vi "merge-array-teste.vi"() -> ()   [LabVIEW 2014]
panel:
  out "output array":dbl[][](array[numeric])=[[49229.86363636363, 160793.81818181818, 459.7801430124, 626.2382997563999, 1419.6569638843712, 2545.9781193333406, 0.005163496779999999], [49166.0, 160790.5, 459.7801430124, 626.2382997563999, 1416.8691367377512, 2555.19013913818, 0.005163496779999999], [48661.068181818184, 159414.9659090909, 459.7801430124, 626.2382997563999, 1394.3056048740445, 2530.385783266425, 0.005163496779999999], [48702.0, 159927.9, 459.7801430124, 626.9865226475, 1405.3506776205356, 2522.9374551760125, 0.005163496779999999], [49455.07575757576, 161404.96212121213, 459.7801430124, 626.2382997563999, 1427.5985476418132, 2551.9671860210565, 0.005163496779999999]]
  in  "Power Meter":dbl[](array[numeric])=[0.005163496779999999, 0.005163496779999999, 0.005163496779999999, 0.005163496779999999, 0.005163496779999999]
  in  "Amplitudes":dbl[][](array[numeric])=[[1419.6569638843712, 2545.9781193333406], [1416.8691367377512, 2555.19013913818], [1394.3056048740445, 2530.385783266425], [1405.3506776205356, 2522.9374551760125], [1427.5985476418132, 2551.9671860210565]]
  in  "Locations Peaks":dbl[][](array[numeric])=[[459.7801430124, 626.2382997563999], [459.7801430124, 626.2382997563999], [459.7801430124, 626.2382997563999], [459.7801430124, 626.9865226475], [459.7801430124, 626.2382997563999]]
  in  "Integration":dbl[][](array[numeric])=[[49229.86363636363, 160793.81818181818], [49166.0, 160790.5], [48661.068181818184, 159414.9659090909], [48702.0, 159927.9], [49455.07575757576, 161404.96212121213]]
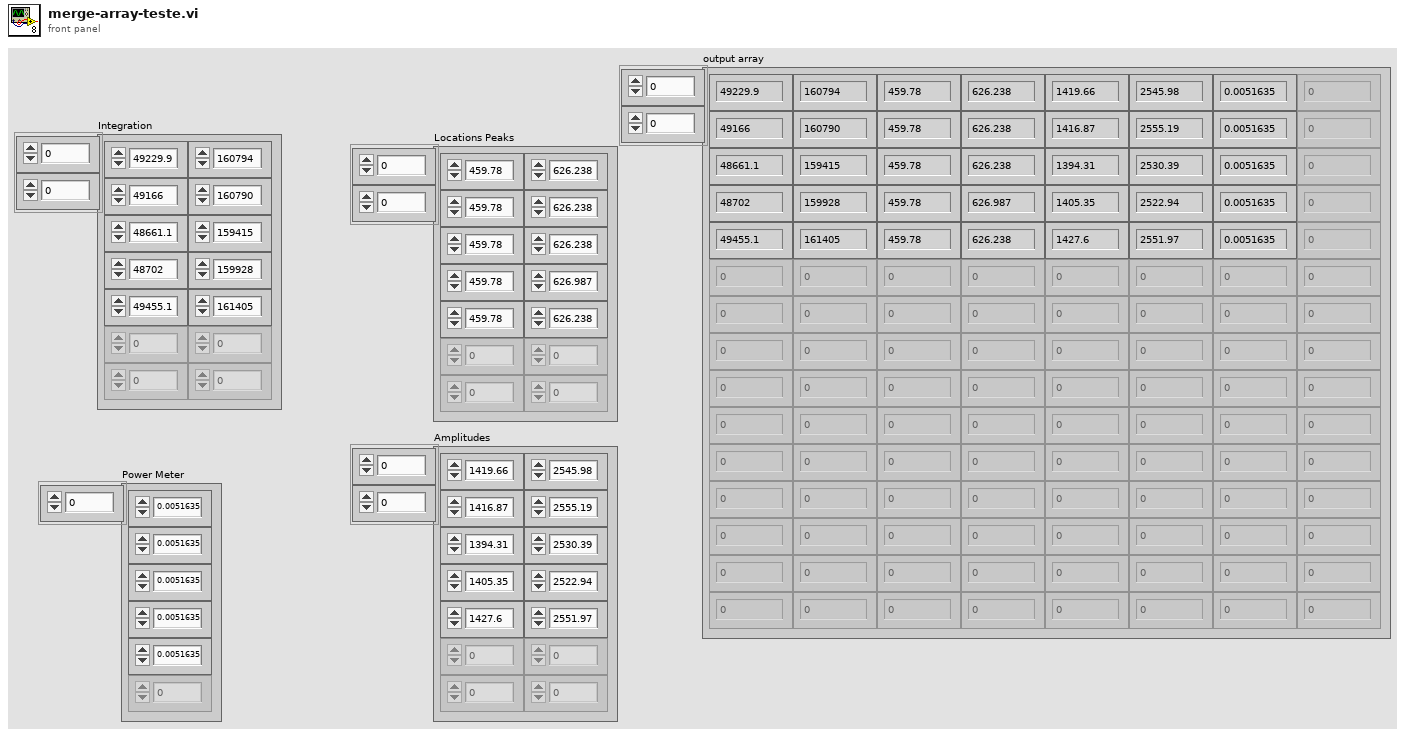
[diagram p1: front panel]
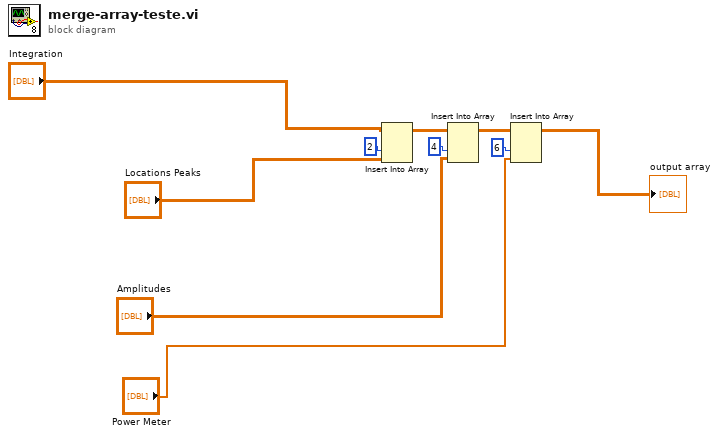
[diagram p0: block diagram]
diagram:
  n1 = Insert Into Array(array="Integration", index (col)=2 ("disabled index (col)"), new element="Locations Peaks") -> (w7:dbl[][])  [unwired: 1 in]
  n2 = Insert Into Array(array=w7, index (col)=4 ("disabled index (col)"), new element="Amplitudes") -> (w2:dbl[][])  [unwired: 1 in]
  n3 = Insert Into Array(array=w2, index (col)=6, new element="Power Meter") -> (→"output array":dbl[][])  [unwired: 1 in]
